vi "WSTRING Byte Stream to String.vi"(8 "error in (no error)":errorcluster, 10 "Byte Stream":u8[](array[numeric])) -> (0 "error out":errorcluster, 2 "Value":string)   [LabVIEW 2018, in "TwinCAT ADS.lvclass"]
uses:
  TwinCAT ADS.lvclass
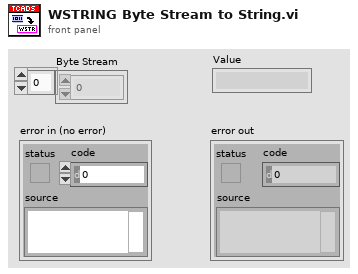
[diagram p1: front panel]
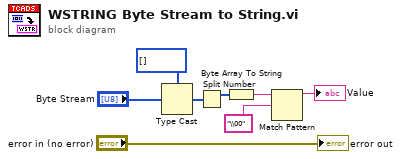
[diagram p0: block diagram]
diagram:
  n1 = Type Cast(type=u16[] [] ("Byte Stream"), x="Byte Stream") -> (*(type *) &x=w4:u16[])
  n2 = Split Number(x=w4) -> (hi(x)=w5:u8[])  [unwired: 1 out]
  n3 = Byte Array To String(unsigned byte array=w5) -> (string=w6:string)
  n4 = Match Pattern(string=w6, regular expression="\\00") -> (before substring=→"Value":string)  [unwired: 1 in, 3 out]
  "error out" <- "error in (no error)"
